vi "Filter Property Tree_MAIN.vi"(7 "Action":T3, 10 "Filter":T1, 11 "Properties for Tree In":T2(array[cluster])) -> (2 "Disabled?":bool[](array[boolean]), 3 "Tree Arr":T4(array[cluster]))   [LabVIEW 2023]
uses:
  controls/action enum.ctl
  <userlib>/_OpenG.lib/comparison/comparison.llb/String Changed__ogtk.vi
  <userlib>/_OpenG.lib/comparison/comparison.llb/Variant Changed__ogtk.vi
panel:
  out "exe time (ms)":u32
  # "Contains only filtered items"
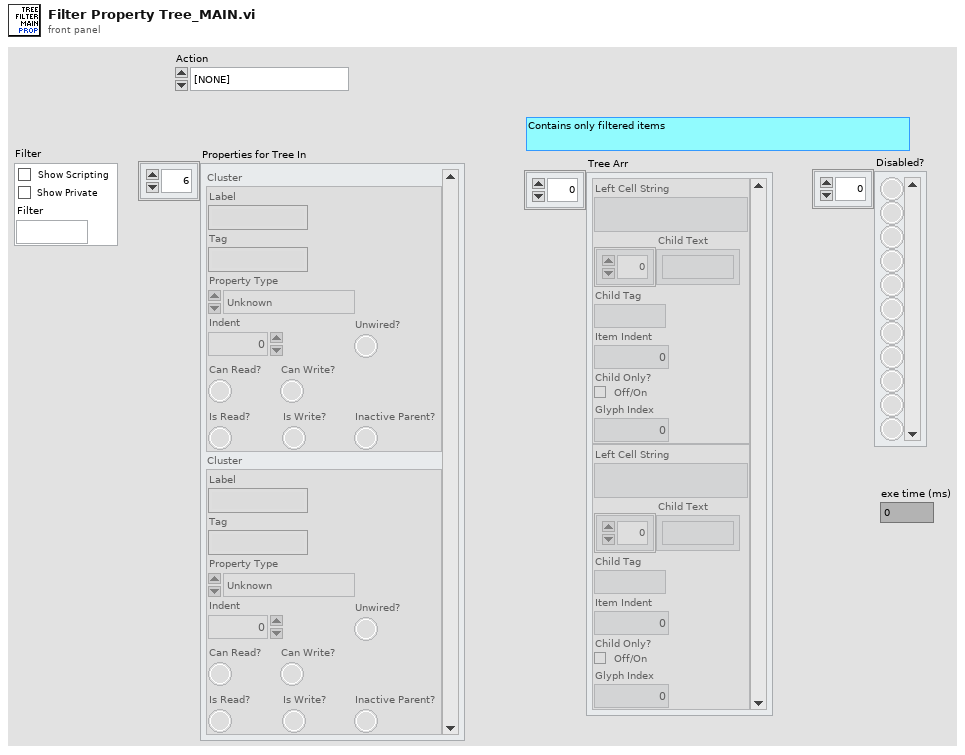
[diagram p1: front panel]
types:
  T1 = cluster{"Show":cluster{"Show Scripting":bool, "Show Private":bool}, "Filter":string}
  T2 = cluster{"Label":string, "Tag":string, "Property Type":enum16{"Unknown", "Base", "Scripting", "Private", "Deprecated", "None", "Divider"}, "Indent":u16, "Can Read?":bool, "Can Write?":bool, "Is Read?":bool, "Is Write?":bool, "Inactive Parent?":bool, "Unwired?":bool}[]
  T3 = typedef "action enum.ctl" = enum16{"[NONE]", "Wire Bundle", "Wire Unbundle", "Terminal Unbundle", "Terminal Bundle", "Bundler Move Up", "Bundler Move Down", "Bundler Insert", "Bundler Remove", "Bundler Remove Unwired", "Bundler Rearrange", "In Place Insert", "In Place Remove", "In Place Remove Unwired", "In Place Rearrange", "Wire Properties", "Wire Method", "Terminal Properties", "Terminal Method", "Property Move Up", "Property Move Down", "Properties Insert", "Properties Remove", "Properties Remove Unwired", "Properties Rearrange", "Method Change", "Class for Constant", "Class For Control", "Class For Node", "Class Name to Clipboard"}
  T4 = cluster{"Left Cell String":string, "Child Text":string[], "Child Tag":string, "Item Indent":i32, "Child Only?":bool, "Glyph Index":i32}[]
  T5 = cluster{"Show Scripting":bool, "Show Private":bool}
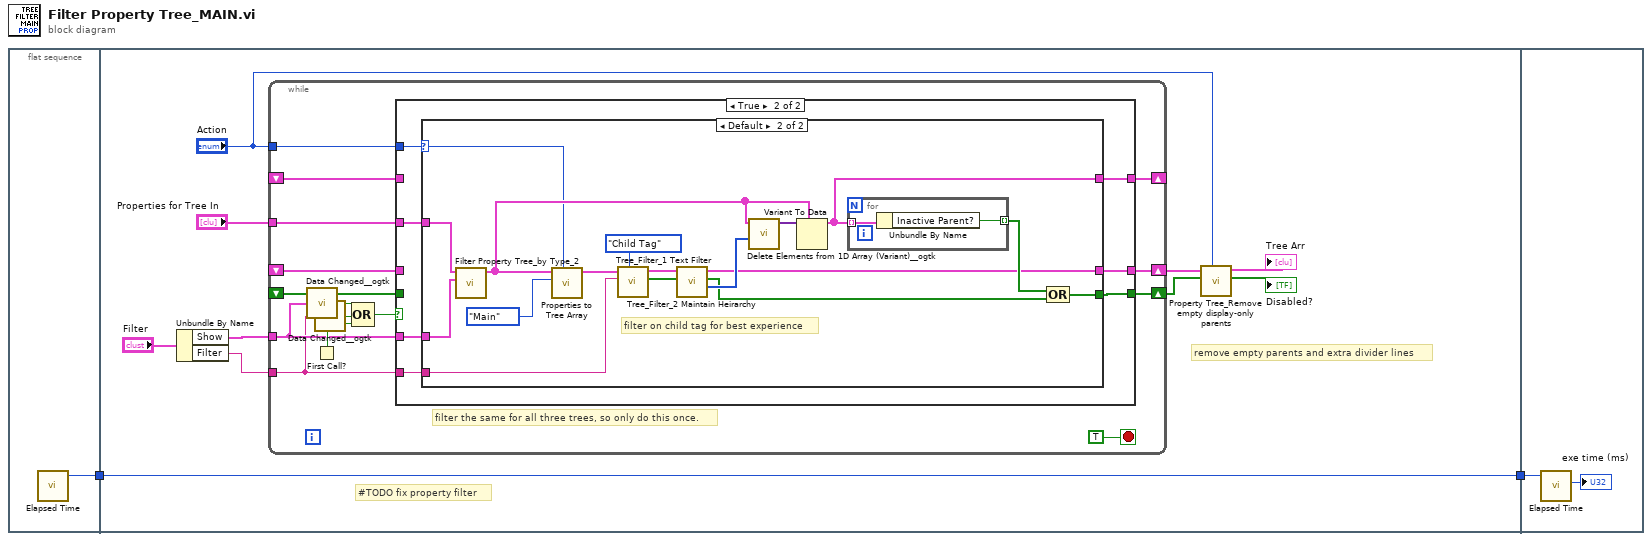
[diagram p0: block diagram]
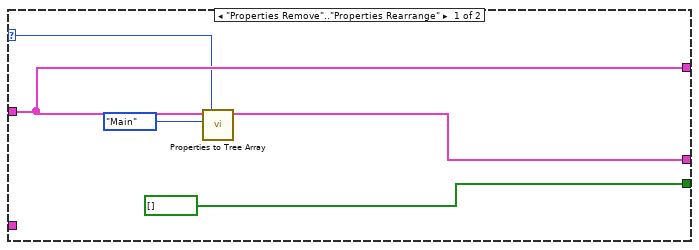
[diagram p3: hidden frame]
diagram:
  n1 = flat-sequence {
    tunnel: [w3] -> w2
    tunnel: w2 -> [w13]
    tunnel: [w13] -> w1
    tunnel: w1 -> [w64]
    frame #0 {
      n2 = call "Elapsed Time.vi"() -> ("millisecond timer value"=w3:u32)  [unwired: 8 in, 3 out]
    }
    frame #1 {
      # "#TODO fix property filter"
      # "remove empty parents and extra divider lines"
      n3 = Unbundle By Name("Filter") -> ("Show"=w11:T5, "Filter"=w10:string)
      n4 = while {
        tunnel: "Action" -> [w28]
        tunnel: "Properties for Tree In" -> [w25]
        tunnel: w11 -> [w15]
        tunnel: w10 -> [w14]
        shift-right: [w27] -> w7
        shift-left: _ -> [w23]
        shift-right: [w26] -> w8
        shift-left: _ -> [w22]
        shift-right: [w19] -> _
        shift-left: _ -> [w18]
        stop <- TRUE stop-if-true
        # "filter the same for all three trees, so only do this once."
        n5 = call-poly <userlib>:"Data Changed__ogtk.vi"("Variant"=w15) -> ("Changed"=w17:bool)
        n6 = First Call?() -> (First Call?: T/F=w21:bool)
        n7 = call-poly <userlib>:"Data Changed__ogtk.vi"("String"=w14) -> ("Changed"=w16:bool)
        n8 = Compound Arithmetic op=OR(w17, w16, w21) -> (w24:bool)
        n9 = case shown="True" w24 {
          tunnel: w28 -> [_ w38]
          tunnel: [w31 w37] -> w27
          tunnel: [w30 w36] -> w26
          tunnel: w25 -> [_ w35]
          tunnel: w15 -> [_ w34]
          tunnel: w14 -> [_ w33]
          tunnel: w23 -> [w31 _]
          tunnel: w22 -> [w30 _]
          tunnel: [w29 w32] -> w19
          tunnel: w18 -> [w29 _]
          frame False {
          }
          frame True {
            n10 = case shown="Default" w38 {
              selector: w38 -> [w40 w45]
              tunnel: [w41 w50] -> w37
              tunnel: [bool[] [] ("Retained Items") w53] -> w36
              tunnel: w35 -> [w42 w51]
              tunnel: w34 -> [_ w49]
              tunnel: w33 -> [_ w48]
              tunnel: [w42 w47] -> w32
              frame "Properties Remove".."Properties Rearrange" {
                n11 = call "Properties to Tree Array.vi"("Action"=w40, "Tree Type"=enum16{"Main", "Write", "Read"}."Main", "Properties for Tree"=w42) -> ("Tree Arr"=w41:T4)  [unwired: 8 in]
              }
              frame Default {
                # "filter on child tag for best experience"
                n12 = call "Filter Property Tree_by Type_2.vi"("Show"=w49, "Properties for Tree"=w51) -> ("Properties for Tree"=w52:T2)  [unwired: 8 in, 1 out]
                n13 = call "Properties to Tree Array.vi"("Action"=w45, "Tree Type"=enum16{"Main", "Write", "Read"}."Main", "Properties for Tree"=w52) -> ("Tree Arr"=w46:T4)  [unwired: 8 in]
                n14 = call "Tree_Filter_1 Text Filter.vi"("Filter On"=enum16{"Left Cell String", "Child Tag"}."Child Tag", "Filter"=w48, "Tree Array in"=w46) -> ("Keep?"=w58:bool[], "Tree Array out"=w60:T4)  [unwired: 7 in]
                n15 = call "Tree_Filter_2 Maintain Heirarchy.vi"("Filter keeps"=w58, "Full Tree Array"=w60) -> ("Incices removed"=w57:i32[], "Retained Items"=w55:bool[], "Tree Array out"=w50:T4)  [unwired: 7 in]
                n16 = call <userlib>:"Delete Elements from 1D Array (Variant)__ogtk.vi"("indices"=w57, "array"=w52) -> ("array w/ subset deleted"=w56:variant[])  [unwired: 8 in, 1 out]
                n17 = Variant To Data(type=w52, Variant=w56) -> (data=w47:T2)  [unwired: 1 in, 1 out]
                n18 = for {
                  tunnel: w47 -> [w62] mode=indexing
                  tunnel: [w61] -> w54 mode=indexing
                  n19 = Unbundle By Name(w62) -> ("Inactive Parent?"=w61:bool)
                }
                n20 = Compound Arithmetic op=OR(w54, w55) -> (w53:bool[])
              }
            }
          }
        }
      }
      n21 = call "Property Tree_Remove empty display-only parents.vi"("Action"="Action", "Disabled?"=w8, "Tree Arr"=w7) -> ("Disabled? Out"=→"Disabled?":bool[], "Tree Arr Out"=→"Tree Arr":T4)  [unwired: 7 in]
    }
    frame #2 {
      n22 = call "Elapsed Time.vi"("past time"=w64) -> ("elapsed time (ms)"=→"exe time (ms)":u32)  [unwired: 7 in, 3 out]
    }
  }
